vi "Trav_Cluster_to_Row.vi"(4 "Traverse line in":T1 {"Row Duration (mins)" format="%#.1f"; "Row No" min=0; "Trace Gas Concentration (%)" min=0.0 format="%#.2f"; "Emission Rate (l/min)" format="%#.2f"; "Tunnel Speed" format="%#.2f"; "Start X" format="%#.2f"; "Start Y" format="%#.2f"; "Start Z" format="%#.2f"; "End X" format="%#.2f"; "End Y" format="%#.2f"; "End Z" format="%#.2f"; "Averaging time (min)" min=0.0 format="%#.2f"}, 6 "Row Number":i32, 7 "Channel names":string[](array[string])) -> (0 "Traverse line Out":T1 {"Row Duration (mins)" format="%#.1f"; "Row No" min=0; "Trace Gas Concentration (%)" min=0.0 format="%#.2f"; "Emission Rate (l/min)" format="%#.2f"; "Tunnel Speed" format="%#.2f"; "Start X" format="%#.2f"; "Start Y" format="%#.2f"; "Start Z" format="%#.2f"; "End X" format="%#.2f"; "End Y" format="%#.2f"; "End Z" format="%#.2f"; "Averaging time (min)" min=0.0 format="%#.2f"}, 1 "Channel Values Out":string[](array[string]))   [LabVIEW 2013]
uses:
  Traverse_cluster.ctl
  Spacing.ctl
  Controls/Multi_run_mode.ctl
  Globals/Trav_pos_global.vi
  Globals/Meas_global.vi
panel:
  # "X           Y            Z"
  # "Start"
  # "End"
  # "X           Y            Z"
  # "Start"
  # "End"
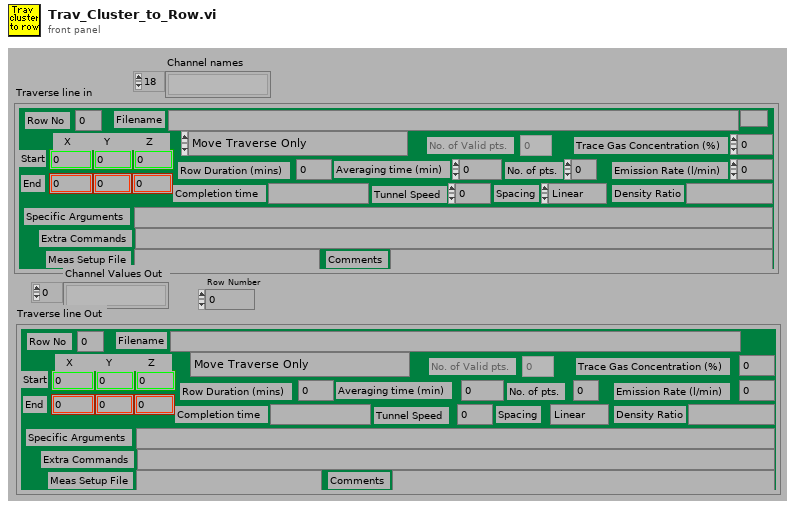
[diagram p1: front panel]
types:
  T1 = typedef "Traverse_cluster.ctl" = cluster{"Start X":dbl, "Start Y":dbl, "Start Z":dbl, "End X":dbl, "End Y":dbl, "End Z":dbl, "No. of pts.":i32, "Spacing":T2, "Filename":path, "Tunnel Speed":dbl, "Averaging time (min)":dbl, "Extra Commands":string, "Specific Arguments":string, "Emission Rate (l/min)":dbl, "Trace Gas Concentration (%)":dbl, "Density Ratio":string, "Comments":string, "Row No":i32, "Row Type Selector":T3, "Completion time":string, "Row Duration (mins)":dbl, "No. of Valid pts.":i32, "Meas Setup File":string}
  T2 = typedef "Spacing.ctl" = enum16{"Linear", "Log", "Gauss", "Specified", "N/A"}
  T3 = typedef "Multi_run_mode.ctl" = enum16{"Move Traverse Only", "Set Tunnel Speed Only", "Set Source Only", "Set Measurement Conditions", "Single Measurement", "Vertical Profile", "Lateral Profile", "Longitudinal Profile", "Explore Volume", "Multi-Axis Profile", "Auto Calibrate", "Meas Fast FID Bkgnd", "Check Beam Power", "Scanning Valve Measurement", "Run VI Named:", "Set ADAM Ch", "Wait (minutes)", "Send Message", "Synchronize With:", "Fall Back to this Row", "Turn Off Row Repeating", "Blank Row", "Traverse 3D Volume"}
  T4 = enum16{"All Channel Names", "Valid Channel Names"}
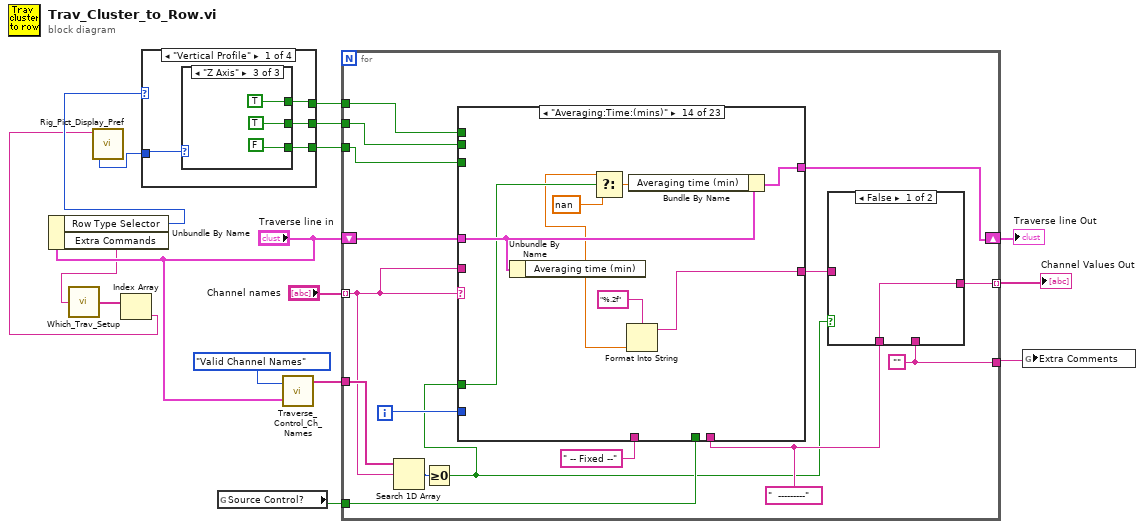
[diagram p0: block diagram]
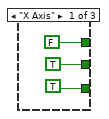
[diagram p2: hidden frame]
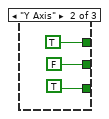
[diagram p3: hidden frame]
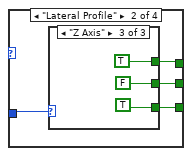
[diagram p4: hidden frame]
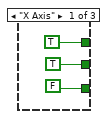
[diagram p5: hidden frame]
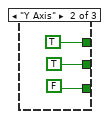
[diagram p6: hidden frame]
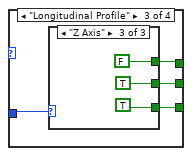
[diagram p7: hidden frame]
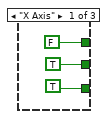
[diagram p8: hidden frame]
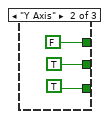
[diagram p9: hidden frame]
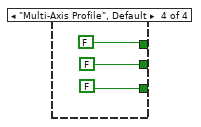
[diagram p10: hidden frame]
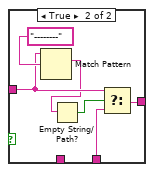
[diagram p11: hidden frame]
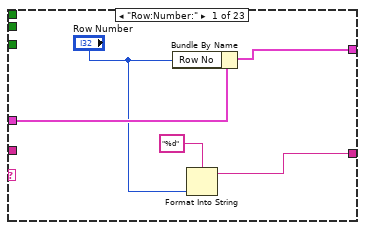
[diagram p12: hidden frame]
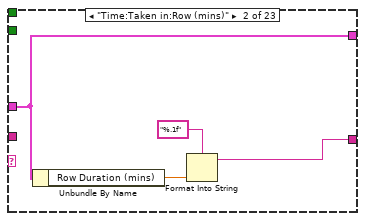
[diagram p13: hidden frame]
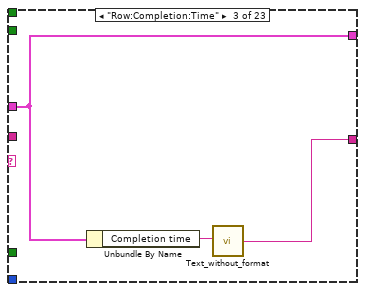
[diagram p14: hidden frame]
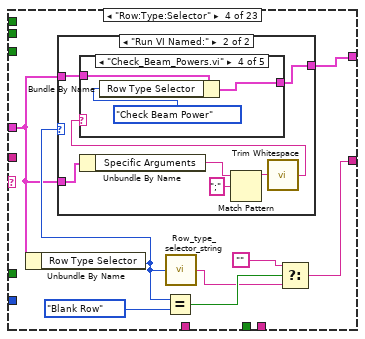
[diagram p15: hidden frame]
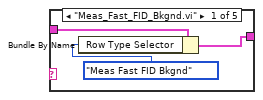
[diagram p17: hidden frame]
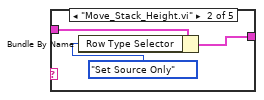
[diagram p18: hidden frame]
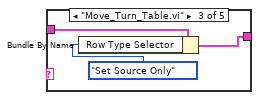
[diagram p19: hidden frame]
diagram:
  n1 = Unbundle By Name("Traverse line in") -> ("Row Type Selector"=w8:T3, "Extra Commands"=w3:string)
  n2 = call "Which_Trav_Setup.vi"("Extra Command String"=w3) -> ("Traverse Setups"=w2:string[])
  n3 = Index Array(array=w2) -> (element=w1:string)  [unwired: 1 in]
  n4 = call "Rig_Pict_Display_Pref.vi"("Traverse Name"=w1) -> ("Which Axis is vertical?"=w9:enum16{"X Axis", "Y Axis", "Z Axis"})  [unwired: 7 out]
  n5 = case shown="\"Vertical Profile\"" w8 {
    tunnel: [w20 w33 w46 FALSE] -> w7
    tunnel: [w19 w32 w45 FALSE] -> w6
    tunnel: [w18 w31 w44 FALSE] -> w5
    tunnel: w9 -> [w17 w30 w43 _]
    frame "Vertical Profile" {
      n6 = case shown="\"Z Axis\"" w17 {
        tunnel: [FALSE TRUE TRUE] -> w20
        tunnel: [TRUE FALSE TRUE] -> w19
        tunnel: [TRUE TRUE FALSE] -> w18
        frame "X Axis" {
        }
        frame "Y Axis" {
        }
        frame "Z Axis" {
        }
      }
    }
    frame "Lateral Profile" {
      n7 = case shown="\"Z Axis\"" w30 {
        tunnel: [TRUE TRUE TRUE] -> w33
        tunnel: [TRUE TRUE FALSE] -> w32
        tunnel: [FALSE FALSE TRUE] -> w31
        frame "X Axis" {
        }
        frame "Y Axis" {
        }
        frame "Z Axis" {
        }
      }
    }
    frame "Longitudinal Profile" {
      n8 = case shown="\"Z Axis\"" w43 {
        tunnel: [FALSE FALSE FALSE] -> w46
        tunnel: [TRUE TRUE TRUE] -> w45
        tunnel: [TRUE TRUE TRUE] -> w44
        frame "X Axis" {
        }
        frame "Y Axis" {
        }
        frame "Z Axis" {
        }
      }
    }
    frame "Multi-Axis Profile", Default {
    }
  }
  n9 = global read "Trav_pos_global.vi" "Source Control?"() -> (w13:bool)
  n10 = call "Traverse_Control_Ch_Names.vi"("Traverse line"="Traverse line in", "Mode"=T4."Valid Channel Names") -> ("Channel names"=w14:string[])
  n11 = for {
    tunnel: "Channel names" -> [w72] mode=indexing
    tunnel: [w68] -> w16 mode=indexing
    shift-right: [w64] -> w10
    shift-left: "Traverse line in" -> [w74]
    tunnel: w14 -> [w73]
    tunnel: w13 -> [w70]
    tunnel: [w65] -> w11
    tunnel: w7 -> [w62]
    tunnel: w6 -> [w60]
    tunnel: w5 -> [w59]
    i -> [w69]
    w65 = ""
    w66 = "  ---------" ("f")
    n12 = Search 1D Array(1D array=w73, element=w72) -> (index of element=w71:i32)  [unwired: 1 out]
    n13 = Greater Or Equal To 0?(x=w71) -> (x >= 0?=w63:bool)
    n14 = case shown="\"Averaging:Time:(mins)\"" w72 {
      tunnel: w74 -> [w83 w87 w93 w94 w128 w137 w144 w153 w164 w175 w186 w192 w199 w214 w226 w228 w245 w255 w266 w273 w286 w296 w298]
      tunnel: [w85 w89 w91 w98 w127 w135 w143 w151 w160 w170 w181 w194 w200 w216 w220 w229 w237 w252 w263 w270 w279 w289 ""] -> w67
      tunnel: w72 -> [_ _ _ _ _ _ _ _ _ _ _ _ _ _ _ _ _ _ _ _ _ _ w300]
      tunnel: [w84 w87 w93 w95 w129 w136 w145 w152 w163 w174 w185 w193 w197 w215 w225 w235 w244 w256 w267 w276 w287 w297 w298] -> w64
      tunnel: w70 -> [_ _ _ _ _ _ _ _ _ _ _ _ _ _ _ _ _ w254 w264 w275 _ _ _]
      tunnel: w69 -> [_ _ _ _ _ _ _ _ _ _ _ _ _ _ _ _ _ _ _ _ _ _ _]
      tunnel: w66 -> [_ _ _ _ _ _ _ _ _ _ _ _ _ _ w222 w227 w239 w251 w262 w271 w280 w290 _]
      tunnel: w63 -> [_ _ _ _ w125 w133 w139 w148 w158 w168 w179 w190 w196 w212 w223 w231 w240 w249 w260 w272 w282 w292 _]
      tunnel: w62 -> [_ _ _ _ _ _ _ _ w162 _ _ _ _ _ _ _ _ _ _ _ _ _ _]
      tunnel: " -- Fixed --" ("t") -> [_ _ _ _ _ _ _ _ w159 w173 w183 _ _ _ _ _ _ _ _ _ _ _ _]
      tunnel: w60 -> [_ _ _ _ _ _ _ _ _ w172 _ _ _ _ _ _ _ _ _ _ _ _ _]
      tunnel: w59 -> [_ _ _ _ _ _ _ _ _ _ w184 _ _ _ _ _ _ _ _ _ _ _ _]
      frame "Row:Number:" {
        n15 = Bundle By Name(cluster=w83, "Row No"="Row Number") -> (w84:T1)
        n16 = Format Into String(format string="%d", "Row Number") -> (resulting string=w85:string)  [unwired: 2 in, 1 out]
      }
      frame "Time:Taken in:Row (mins)" {
        n17 = Unbundle By Name(w87) -> ("Row Duration (mins)"=w88:dbl)
        n18 = Format Into String(format string="%.1f", w88) -> (resulting string=w89:string)  [unwired: 2 in, 1 out]
      }
      frame "Row:Completion:Time" {
        n19 = Unbundle By Name(w93) -> ("Completion time"=w92:string)
        n20 = call "Text_without_format.vi"("Input string"=w92) -> ("Output string"=w91:string)
      }
      frame "Row:Type:Selector" {
        n21 = Unbundle By Name(w94) -> ("Row Type Selector"=w96:T3)
        n22 = case shown="\"Run VI Named:\"" w96 {
          tunnel: w94 -> [_ w109]
          tunnel: [w102 w108] -> w95
          tunnel: w94 -> [w102 w107]
          frame "Move Traverse Only", Default {
          }
          frame "Run VI Named:" {
            n23 = Unbundle By Name(w109) -> ("Specific Arguments"=w105:string)
            n24 = Match Pattern(string=w105, regular expression=";") -> (before substring=w104:string)  [unwired: 4 out]
            n25 = call <vilib>:"Trim Whitespace.vi"("string"=w104) -> ("trimmed string"=w103:string)  [unwired: 1 in]
            n26 = case shown="\"Check_Beam_Powers.vi\"" w103 {
              tunnel: [w110 w113 w116 w119 w122] -> w108
              tunnel: w107 -> [w112 w114 w117 w120 w122]
              frame "Meas_Fast_FID_Bkgnd.vi" {
                n27 = Bundle By Name(cluster=w112, "Row Type Selector"=Multi_run_mode."Meas Fast FID Bkgnd" ("Mode")) -> (w110:T1)
              }
              frame "Move_Stack_Height.vi" {
                n28 = Bundle By Name(cluster=w114, "Row Type Selector"=Multi_run_mode."Set Source Only" ("Mode")) -> (w113:T1)
              }
              frame "Move_Turn_Table.vi" {
                n29 = Bundle By Name(cluster=w117, "Row Type Selector"=Multi_run_mode."Set Source Only" ("Mode")) -> (w116:T1)
              }
              frame "Check_Beam_Powers.vi" {
                n30 = Bundle By Name(cluster=w120, "Row Type Selector"=Multi_run_mode."Check Beam Power" ("Mode")) -> (w119:T1)
              }
              frame "No Match", Default {
              }
            }
          }
        }
        n31 = Equal?(x=w96, y=Multi_run_mode."Blank Row" ("Mode")) -> (x = y?=w100:bool)
        n32 = call "Row_type_selector_string.vi"("Mode"=w96) -> ("Output string"=w99:string)
        n33 = Select(t="", s=w100, f=w99) -> (s? t:f=w98:string)
      }
      frame "Tunnel:Speed:(m/s)" {
        n34 = Unbundle By Name(w128) -> ("Tunnel Speed"=w124:dbl)
        n35 = Select(t=w124, s=w125, f=nan) -> (s? t:f=w123:dbl)
        n36 = Bundle By Name(cluster=w128, "Tunnel Speed"=w123) -> (w129:T1)
        n37 = Format Into String(format string="%f", w124) -> (resulting string=w127:string)  [unwired: 2 in, 1 out]
      }
      frame "Start at:X:(mm)" {
        n38 = Unbundle By Name(w137) -> ("Start X"=w131:dbl)
        n39 = Select(t=w131, s=w133, f=nan) -> (s? t:f=w132:dbl)
        n40 = Format Into String(format string="%.3f", w131) -> (resulting string=w135:string)  [unwired: 2 in, 1 out]
        n41 = Bundle By Name(cluster=w137, "Start X"=w132) -> (w136:T1)
      }
      frame "Start at:Y:(mm)" {
        n42 = Unbundle By Name(w144) -> ("Start Y"=w140:dbl)
        n43 = Select(t=w140, s=w139, f=nan) -> (s? t:f=w141:dbl)
        n44 = Format Into String(format string="%.3f", w140) -> (resulting string=w143:string)  [unwired: 2 in, 1 out]
        n45 = Bundle By Name(cluster=w144, "Start Y"=w141) -> (w145:T1)
      }
      frame "Start at:Z:(mm)" {
        n46 = Unbundle By Name(w153) -> ("Start Z"=w149:dbl)
        n47 = Select(t=w149, s=w148, f=nan) -> (s? t:f=w147:dbl)
        n48 = Bundle By Name(cluster=w153, "Start Z"=w147) -> (w152:T1)
        n49 = Format Into String(format string="%.3f", w149) -> (resulting string=w151:string)  [unwired: 2 in, 1 out]
      }
      frame "End at:X:(mm)" {
        n50 = Unbundle By Name(w164) -> ("End X"=w155:dbl)
        n51 = Format Into String(format string="%.3f", w155) -> (resulting string=w161:string)  [unwired: 2 in, 1 out]
        n52 = Select(t=w155, s=w158, f=nan) -> (s? t:f=w156:dbl)
        n53 = Bundle By Name(cluster=w164, "End X"=w156) -> (w163:T1)
        n54 = Select(t=w159, s=w162, f=w161) -> (s? t:f=w160:string)
      }
      frame "End at:Y:(mm)" {
        n55 = Unbundle By Name(w175) -> ("End Y"=w167:dbl)
        n56 = Select(t=w167, s=w168, f=nan) -> (s? t:f=w166:dbl)
        n57 = Bundle By Name(cluster=w175, "End Y"=w166) -> (w174:T1)
        n58 = Format Into String(format string="%.3f", w167) -> (resulting string=w171:string)  [unwired: 2 in, 1 out]
        n59 = Select(t=w173, s=w172, f=w171) -> (s? t:f=w170:string)
      }
      frame "End at:Z:(mm)" {
        n60 = Unbundle By Name(w186) -> ("End Z"=w178:dbl)
        n61 = Select(t=w178, s=w179, f=nan) -> (s? t:f=w177:dbl)
        n62 = Bundle By Name(cluster=w186, "End Z"=w177) -> (w185:T1)
        n63 = Format Into String(format string="%.3f", w178) -> (resulting string=w182:string)  [unwired: 2 in, 1 out]
        n64 = Select(t=w183, s=w184, f=w182) -> (s? t:f=w181:string)
      }
      frame "Number:Of:Points" {
        n65 = Unbundle By Name(w192) -> ("No. of pts."=w188:i32)
        n66 = Format Into String(format string="%d", w188) -> (resulting string=w194:string)  [unwired: 2 in, 1 out]
        n67 = Select(t=w188, s=w190, f=0 ("t")) -> (s? t:f=w191:i32)
        n68 = Bundle By Name(cluster=w192, "No. of pts."=w191) -> (w193:T1)
      }
      frame "Point:Spacing:Method" {
        n69 = Unbundle By Name(w199) -> ("Spacing"=w198:T2)
        n70 = case shown="\"N/A\"" w198 {
          tunnel: ["Linear" "Log" "Gauss" "Specified" "N/A"] -> w200
          frame "Linear" {
          }
          frame "Log" {
          }
          frame "Gauss" {
          }
          frame "Specified" {
          }
          frame "N/A" {
          }
        }
        n71 = case shown="True" w196 {
          tunnel: w199 -> [w203 w204]
          tunnel: [w201 w204] -> w197
          frame False {
            n72 = Bundle By Name(cluster=w203, "Spacing"=Spacing."N/A") -> (w201:T1)
          }
          frame True {
          }
        }
      }
      frame "Averaging:Time:(mins)" {
        n73 = Unbundle By Name(w214) -> ("Averaging time (min)"=w210:dbl)
        n74 = Select(t=w210, s=w212, f=nan) -> (s? t:f=w211:dbl)
        n75 = Format Into String(format string="%.2f", w210) -> (resulting string=w216:string)  [unwired: 2 in, 1 out]
        n76 = Bundle By Name(cluster=w214, "Averaging time (min)"=w211) -> (w215:T1)
      }
      frame "Filename:HD:Users" {
        n77 = Unbundle By Name(w226) -> ("Filename"=w224:path)
        n78 = Path To String(path=w224) -> (string=w219:string)
        n79 = call "Text_without_format.vi"("Input string"=w219) -> ("Output string"=w220:string)
        n80 = Select(t=w220, s=w223, f=w222) -> (s? t:f=w221:string)
        n81 = String To Path(string=w221) -> (path=w218:path)
        n82 = Bundle By Name(cluster=w226, "Filename"=w218) -> (w225:T1)
      }
      frame "Specific:Arguments:String" {
        n83 = Unbundle By Name(w228) -> ("Specific Arguments"=w236:string)
        n84 = call "Text_without_format.vi"("Input string"=w236) -> ("Output string"=w232:string)
        n85 = Not Equal?(x=w232, y=w227) -> (x != y?=w234:bool)
        n86 = Select(t=w232, s=w234, f="") -> (s? t:f=w229:string)
        n87 = Select(t=w229, s=w231, f=w227) -> (s? t:f=w230:string)
        n88 = Bundle By Name(cluster=w228, "Specific Arguments"=w230) -> (w235:T1)
      }
      frame "Extra:Commands:String" {
        n89 = Unbundle By Name(w245) -> ("Extra Commands"=w246:string)
        n90 = call "Text_without_format.vi"("Input string"=w246) -> ("Output string"=w241:string)
        n91 = Not Equal?(x=w241, y=w239) -> (x != y?=w243:bool)
        n92 = Select(t=w241, s=w243, f="") -> (s? t:f=w237:string)
        n93 = Select(t=w237, s=w240, f=w239) -> (s? t:f=w238:string)
        n94 = Bundle By Name(cluster=w245, "Extra Commands"=w238) -> (w244:T1)
      }
      frame "Emission:Rate:(l/min)" {
        n95 = Unbundle By Name(w255) -> ("Emission Rate (l/min)"=w248:dbl)
        n96 = Select(t=w248, s=w249, f=nan) -> (s? t:f=w247:dbl)
        n97 = Bundle By Name(cluster=w255, "Emission Rate (l/min)"=w247) -> (w256:T1)
        n98 = Format Into String(format string="%.2f", w248) -> (resulting string=w253:string)  [unwired: 2 in, 1 out]
        n99 = Select(t=w253, s=w254, f=w251) -> (s? t:f=w252:string)
      }
      frame "Trace Gas:Concentration:(%)" {
        n100 = Unbundle By Name(w266) -> ("Trace Gas Concentration (%)"=w259:dbl)
        n101 = Select(t=w259, s=w260, f=nan) -> (s? t:f=w258:dbl)
        n102 = Bundle By Name(cluster=w266, "Trace Gas Concentration (%)"=w258) -> (w267:T1)
        n103 = Format Into String(format string="%.3f", w259) -> (resulting string=w265:string)  [unwired: 2 in, 1 out]
        n104 = Select(t=w265, s=w264, f=w262) -> (s? t:f=w263:string)
      }
      frame "Density:Ratio:" {
        n105 = Unbundle By Name(w273) -> ("Density Ratio"=w277:string)
        n106 = call "Text_without_format.vi"("Input string"=w277) -> ("Output string"=w274:string)
        n107 = Select(t=w274, s=w275, f=w271) -> (s? t:f=w270:string)
        n108 = Select(t=w270, s=w272, f=w271) -> (s? t:f=w269:string)
        n109 = Bundle By Name(cluster=w273, "Density Ratio"=w269) -> (w276:T1)
      }
      frame "Comments::" {
        n110 = Unbundle By Name(w286) -> ("Comments"=w278:string)
        n111 = call "Text_without_format.vi"("Input string"=w278) -> ("Output string"=w283:string)
        n112 = Not Equal?(x=w283, y=w280) -> (x != y?=w285:bool)
        n113 = Select(t=w283, s=w285, f="") -> (s? t:f=w279:string)
        n114 = Select(t=w279, s=w282, f=w280) -> (s? t:f=w281:string)
        n115 = Bundle By Name(cluster=w286, "Comments"=w281) -> (w287:T1)
      }
      frame "Measurement:Setup:File" {
        n116 = Unbundle By Name(w296) -> ("Meas Setup File"=w288:string)
        n117 = call "Text_without_format.vi"("Input string"=w288) -> ("Output string"=w293:string)
        n118 = Not Equal?(x=w293, y=w290) -> (x != y?=w295:bool)
        n119 = Select(t=w293, s=w295, f="") -> (s? t:f=w289:string)
        n120 = Select(t=w289, s=w292, f=w290) -> (s? t:f=w291:string)
        n121 = Bundle By Name(cluster=w296, "Meas Setup File"=w291) -> (w297:T1)
      }
      frame "No match", Default {
        n122 = call "Was_string_matched.vi"("Variable name"=w300) -> ()  [unwired: 2 in]
      }
    }
    n123 = case shown="False" w63 {
      tunnel: [w75 w80] -> w68
      tunnel: w67 -> [_ w78]
      tunnel: w66 -> [w75 _]
      tunnel: w65 -> [_ w81]
      frame False {
      }
      frame True {
        n124 = Match Pattern(string=w78, regular expression="--------" ("f")) -> (match substring=w77:string)  [unwired: 4 out]
        n125 = Empty String/Path?(string/path=w77) -> (empty?=w76:bool)
        n126 = Select(t=w78, s=w76, f=w81) -> (s? t:f=w80:string)
      }
    }
  }
  "Channel Values Out" <- w16
  "Traverse line Out" <- w10
  n127 = global write "Meas_global.vi" "Extra Comments"(w11) -> ()
